vi "FPGA_8a_ws.vi"() -> ()   [LabVIEW 2015]
doc: "This VI reads a buffer of single point values from all four channels of the NI 923x and places the acquired data into a DMA FIFO."
uses:
  <vilib>/LabVIEW Targets/FPGA/cRIO/shared/nicrio_ModuleControls/nicrio_cRIO-9234_DataRatesRing2.ctl
  <vilib>/LabVIEW Targets/FPGA/cRIO/shared/nicrio_ModuleControls/nicrio_BasicConversionTime.ctl
  <vilib>/rvi/Emulation/niFpgaGetClockAttributes.vi
  <vilib>/rvi/Emulation/niFpgaSctlEmulationGetInTimedLoop.vi
  <vilib>/rvi/Emulation/niFpgaEmulationReportErrorSimple.vi
  <vilib>/rvi/eio/common/nirviEmuTemplateMethod_errors.vi
  <vilib>/rvi/Emulation/niFpgaCriticalErrorInLSC.vi
  <vilib>/rvi/eio/common/nirviEmuTemplatePropertySet_errors.vi
  <vilib>/rvi/Emulation/niFpgaProcessEmulError.vi
  <vilib>/rvi/interface/RandomDataEmulation/niFpgaRandomDataHandleErrors.vi
  <vilib>/eio/EIONode/EIONode.xnode
  <vilib>/eio/EIOPropertyNode/EIOPropertyNode.xnode
  <vilib>/rvi/DataTransferAndStorage/Container/XNode/niFpgaContainer.xnode
  <vilib>/rvi/interface/RandomDataEmulation/nirviRandomDataFpgaReadWriteTemplate.vi
  <vilib>/rvi/eio/common/nirviEmuTemplatePropertyGet_errors.vi
  <vilib>/rvi/eio/common/nirviEmuTemplatePropertyGet_noerrors.vi
  <vilib>/rvi/eio/common/nirviEmuTemplatePropertySet_noerrors.vi
panel:
  in  "Digital?":bool=TRUE
  out "Numeric 2":i32
  out "WhlCnt":fxp<+/-,24,-4> format="%.27g"
  in  "Offset_rueda":fxp<+/-,24,-4> format="%.27g"
  out "Rueda?":i16
  in  "Conversion Time":T1
  in  "Canal ccero?":bool=TRUE
  in  "Count(mSec)":u32=2
  out "Chassis Temperature":i16
  out "Fotocelula":bool
  out "Detector de\npresencia":bool
  in  "Fotocélula":bool
  out "DC OK":bool
  in  "Data Rate":T2=2 items=["51.200 kS/s (NI 9234)"=1, "25.600 kS/s (NI 9234)"=2, "17.067 kS/s (NI 9234)"=3, "12.800 kS/s (NI 9234)"=4, "10.240 kS/s (NI 9234)"=5, "8.533 kS/s (NI 9234)"=6, "7.314 kS/s (NI 9234)"=7, "6.400 kS/s (NI 9234)"=8, "5.689 kS/s (NI 9234)"=9, "5.120 kS/s (NI 9234)"=10, "4.654 kS/s (NI 9234)"=11, "4.267 kS/s (NI 9234)"=12, "3.938 kS/s (NI 9234)"=13, "3.657 kS/s (NI 9234)"=14, "3.413 kS/s (NI 9234)"=15, "3.200 kS/s (NI 9234)"=16, "3.012 kS/s (NI 9234)"=17, "2.845 kS/s (NI 9234)"=18, "2.695 kS/s (NI 9234)"=19, "2.560 kS/s (NI 9234)"=20, "2.438 kS/s (NI 9234)"=21, "2.328 kS/s (NI 9234)"=22, "2.226 kS/s (NI 9234)"=23, "2.133 kS/s (NI 9234)"=24, "2.048 kS/s (NI 9234)"=25, "1.969 kS/s (NI 9234)"=26, "1.896 kS/s (NI 9234)"=27, "1.829 kS/s (NI 9234)"=28, "1.765 kS/s (NI 9234)"=29, "1.707 kS/s (NI 9234)"=30, "1.652 kS/s (NI 9234)"=31]
  out "Buffer Overflow":bool
  in  "Stop":bool
  out "Buffer Underflow":bool
  out "Error Out":errorcluster
  # "For instructions, and select Help>>Show Context Help and hover over the icon."
  # "Timing Parameters"
  # "Output Parameters"
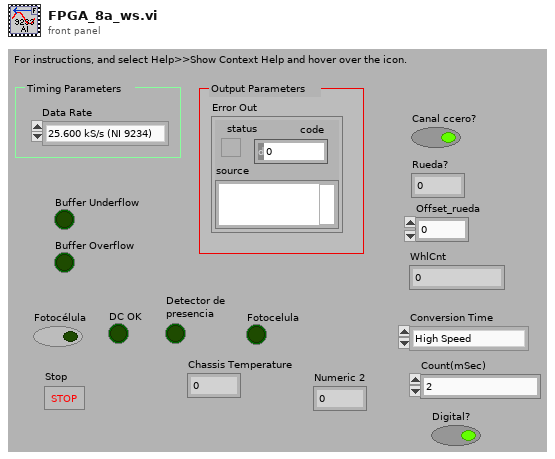
[diagram p1: front panel]
types:
  T1 = typedef "nicrio_BasicConversionTime.ctl" = enum8{"High Speed", "High Resolution"}
  T2 = typedef "nicrio_cRIO-9234_DataRatesRing2.ctl" = u8
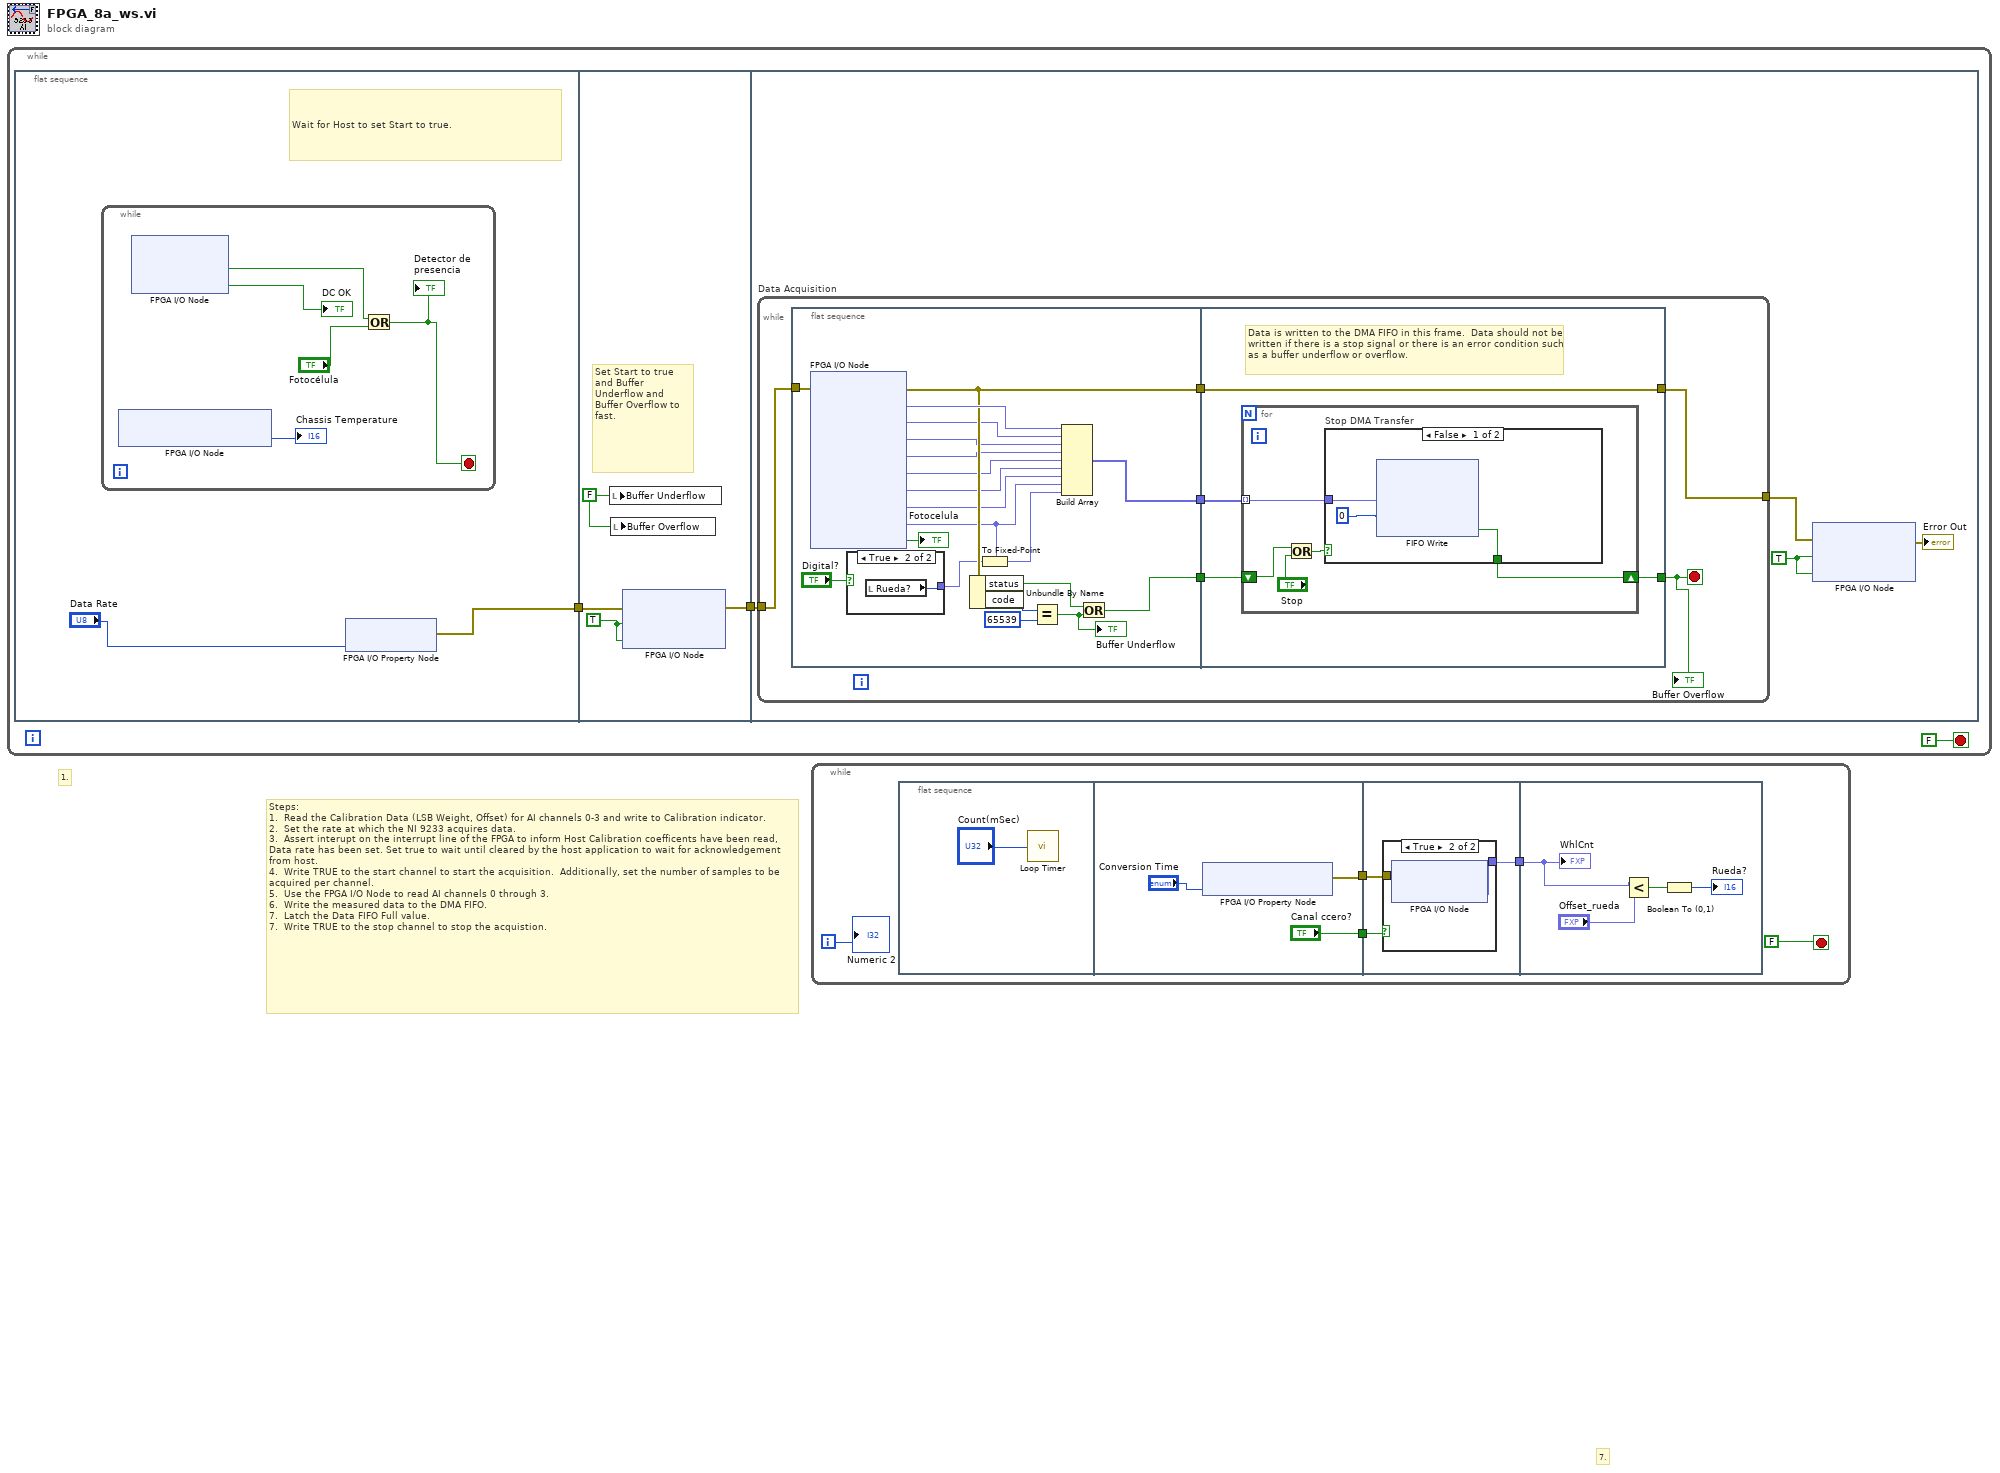
[diagram p0: block diagram]
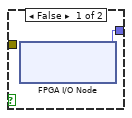
[diagram p2: hidden frame]
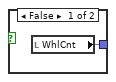
[diagram p3: hidden frame]
diagram:
  # "7."
  # "Steps: \n1.  Read the Calibration Data (LSB Weight, Offset) for AI channels 0-3 and write to Calibration indicator.\n2.  Set the rate at which the NI 9233 acquires data. \n3.  Assert interupt on the interrupt line of the FPGA to inform Host Calibration coefficents have been read, Data rate has been set. Set true to wait until cleared by the host application to wait for acknowledgement from host.\n4.  Write TRUE to the start channel to start the acquisition.  Additionally, set the number of samples to be acquired per channel.\n5.  Use the FPGA I/O Node to read AI channels 0 through 3. \n6.  Write the measured data to the DMA FIFO.\n7.  Latch the Data FIFO Full value.\n7.  Write TRUE to the stop channel to stop the acquistion."
  # "1."
  n1 = while {
    stop <- FALSE stop-if-true
    n2 = flat-sequence "MainSeq" {
      tunnel: [w5] -> w2
      tunnel: w2 -> [w13]
      tunnel: [w12] -> w1
      tunnel: w1 -> [w18]
      frame #0 {
        # "Wait for Host to set Start to true."
        n3 = while "initWait" {
          stop <- w7 stop-if-true
          n4 = xnode "FPGA I/O Node"() -> ("Chassis Temperature"=→"Chassis Temperature":i16)  [unwired: 1 in, 1 out]
          n5 = xnode "FPGA I/O Node"() -> ("Mod3/DI0"=w9:bool, "Mod3/DI2"=→"DC OK":bool)  [unwired: 3 in, 3 out]
          n6 = Or(x=w9, y="Fotocélula") -> (x .or. y?=w7:bool)
          "Detector de\npresencia" <- w7
        }
        n7 = xnode "FPGA I/O Property Node"("Data Rate"="Data Rate") -> ("error out"=w5:errorcluster)  [unwired: 2 in, 1 out]
      }
      frame #1 {
        w11 = TRUE
        w14 = FALSE ("Late? (Latched)")
        # "Set Start to true and Buffer Underflow and Buffer Overflow to fast."
        n8 = local write "Buffer Underflow"(w14) -> ()
        n9 = local write "Buffer Overflow"(w14) -> ()
        n10 = xnode "FPGA I/O Node"("error in"=w13, "Mod1/Start"=w11, "Mod2/Start"=w11) -> ("error out"=w12:errorcluster)  [unwired: 2 in, 2 out]
      }
      frame #2 {
        w15 = TRUE
        n11 = while "Data Acquisition" {
          tunnel: w18 -> [w22]
          tunnel: [w21] -> w16
          stop <- w19 stop-if-true
          n12 = flat-sequence "Data Acquisition Sequence" {
            tunnel: [w43] -> w24
            tunnel: [w34] -> w23
            tunnel: w22 -> [w42]
            tunnel: [w41] -> w20
            tunnel: w24 -> [w50]
            tunnel: w23 -> [w49]
            tunnel: [w48] -> w19
            tunnel: [w47] -> w21
            tunnel: w20 -> [w47]
            frame #0 {
              n13 = xnode "FPGA I/O Node"("error in"=w42) -> ("error out"=w41:errorcluster, "Mod1/AI0"=w44:fxp<+/-,24,4>, "Mod1/AI1"=w37:fxp<+/-,24,4>, "Mod1/AI2"=w36:fxp<+/-,24,4>, "Mod1/AI3"=w35:fxp<+/-,24,4>, "Mod2/AI0"=w32:fxp<+/-,24,4>, "Mod2/AI1"=w31:fxp<+/-,24,4>, "Mod2/AI2"=w30:fxp<+/-,24,4>, "Mod2/AI3"=w28:fxp<+/-,24,4>, "Mod3/DI0"=→"Fotocelula":bool)  [unwired: 9 in, 9 out]
              n14 = case shown="True" "Digital?" {
                tunnel: [w45 w46] -> w25
                frame False {
                  n15 = local read "WhlCnt"() -> (w45:fxp<+/-,24,-4>)
                }
                frame True {
                  n16 = local read "Rueda?"() -> (w46:i16)
                }
              }
              n17 = Unbundle By Name(w41) -> ("status"=w33:bool, "code"=w40:i32)
              n18 = To Fixed-Point(fixed-point type=w28, number=w25) -> (fixed-point=w27:fxp<+/-,24,4>)
              n19 = Equal?(x=w40, y=65539) -> (x = y?=w38:bool)
              "Buffer Underflow" <- w38
              n20 = Build Array(w44, w37, w36, w35, w32, w31, w30, w28, w27) -> (w43:fxp<+/-,24,4>[])
              n21 = Or(x=w33, y=w38) -> (x .or. y?=w34:bool)
            }
            frame #1 {
              # "Data is written to the DMA FIFO in this frame.  Data should not be\nwritten if there is a stop signal or there is an error condition such \nas a buffer underflow or overflow."
              n22 = for "DMAWriteLoop" {
                tunnel: w50 -> [w55] mode=indexing
                shift-right: [w51] -> w48
                shift-left: w49 -> [w53]
                n23 = Or(x=w53, y="Stop") -> (x .or. y?=w52:bool)
                n24 = case "Stop DMA Transfer" shown="False" w52 {
                  selector: w52 -> [_ w59]
                  tunnel: w55 -> [w56 _]
                  tunnel: [w58 w59] -> w51
                  frame False {
                    n25 = xnode ("FIFO Write")("Element"=w56, "Timeout"=0) -> ("Timed Out?"=w58:bool)  [unwired: 1 in, 1 out]
                  }
                  frame True {
                  }
                }
              }
            }
          }
          "Buffer Overflow" <- w19
        }
        n26 = xnode "FPGA I/O Node"("error in"=w16, "Mod1/Stop"=w15, "Mod2/Stop"=w15) -> ("error out"=→"Error Out":errorcluster)  [unwired: 2 in, 2 out]
      }
    }
  }
  n27 = while {
    i -> [w64]
    stop <- FALSE stop-if-true
    n28 = flat-sequence {
      tunnel: [w68] -> w62
      tunnel: ["Canal ccero?"] -> w60
      tunnel: [w71] -> w63
      tunnel: w62 -> [w70]
      tunnel: w60 -> [w69]
      tunnel: w63 -> [w77]
      frame #0 {
        n29 = call "Loop Timer"("Count(mSec)"="Count(mSec)") -> ()  [unwired: 1 out]
      }
      frame #1 {
        n30 = xnode "FPGA I/O Property Node"("Conversion Time"="Conversion Time") -> ("error out"=w68:errorcluster)  [unwired: 2 in, 1 out]
      }
      frame #2 {
        n31 = case shown="True" w69 {
          tunnel: [w72 w74] -> w71
          tunnel: w70 -> [_ w73]
          frame False {
            n32 = xnode "FPGA I/O Node"() -> ("Mod4/AI1"=w72:fxp<+/-,24,-4>)  [unwired: 2 in, 2 out]
          }
          frame True {
            n33 = xnode "FPGA I/O Node"("error in"=w73) -> ("Mod4/AI0"=w74:fxp<+/-,24,-4>)  [unwired: 1 in, 2 out]
          }
        }
      }
      frame #3 {
        n34 = Less?(x=w77, y="Offset_rueda") -> (x < y?=w76:bool)
        n35 = Boolean To (0,1)(Boolean=w76) -> (0, 1=→"Rueda?":i16)
        "WhlCnt" <- w77
      }
    }
    "Numeric 2" <- w64
  }
